vi "Real-Time Main-Final_Local_Digital.vi"() -> ()   [LabVIEW 2024]
uses:
  <vilib>/Platform/TimedLoop/XDataNode/timing_clust.ctl
  <vilib>/Platform/TimedLoop/XDataNode/nitl_modes.ctl
  <vilib>/Platform/TimedLoop/XDataNode/wakeup.ctl
  <instrlib>/niScope/Controls/niScope trigger source digital.ctl
  <instrlib>/niScope/Configure/Trigger/niScope Configure Trigger Digital.vi
  <instrlib>/niScope/Acquire/Fetch/niScope Fetch WDT.vi
  <vilib>/Waveform/WDTOps.llb/WDT Get Waveform Time Array DBL.vi
  <vilib>/platform/TimedLoop/XDataNode/XDataNode.xnode
  <vilib>/Platform/TimedLoop/XDataNode/XDNodeRunTimeDep.lvlib
panel:
  in  "channels":string="0"
  in  "FileName":string
  out "# of Chunks Fetched":i32
  out "# of Points Fetched":i32
  out "Horizontal:Actual Sample Rate":dbl
  in  "stop":bool
  in  "Fetch:Fetch Relative To":i32(ring)=482 items=["Start"=482, "Trigger"=483, "Pretrigger"=477, "Now"=481, "Read Pointer"=388]
  out "wfm":waveform(dbl)(graph)
  out "Time_shift":dbl
  in  "Resource Name":refnum<k15>="Dev1" caption="Resource Name(s)"
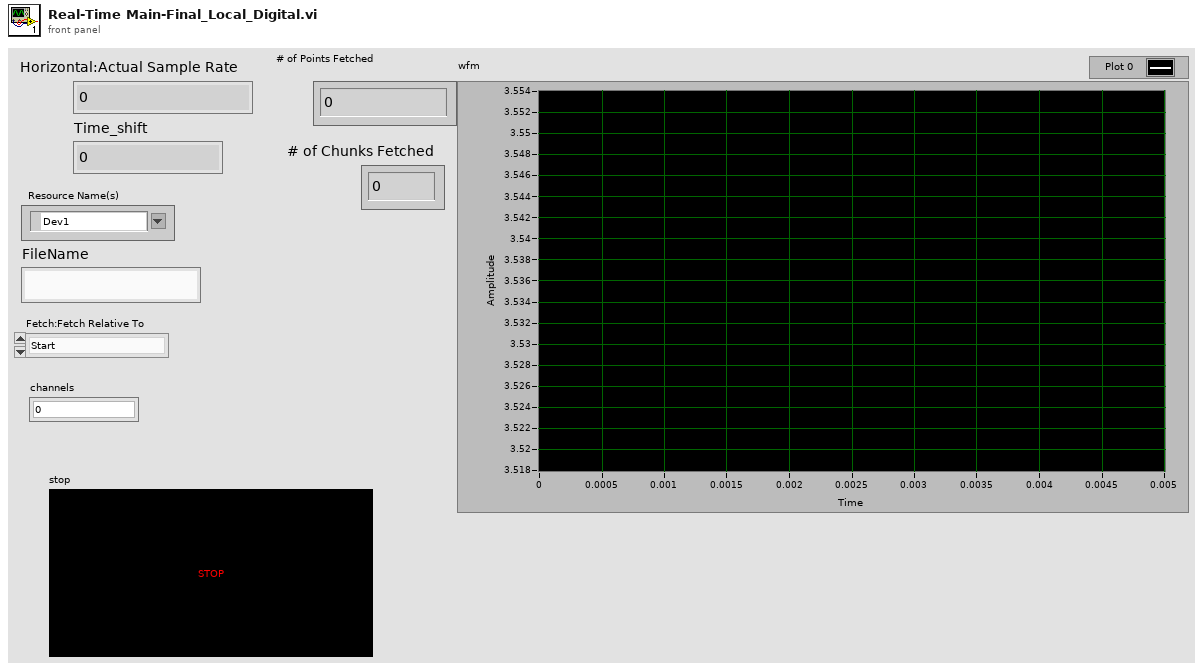
[diagram p1: front panel]
types:
  T1 = enum16{"open", "open or create", "create or replace", "create", "open (read-only)"}
  T2 = typedef "XDNodeRunTimeDep.lvlib/timing_clust.ctl" = cluster{"Expected End [f-1]":u64, "Actual End [f-1]":u64, "Finished Late? [f-1]":bool, "Expected End [i-1]":u64, "Actual End [i-1]":u64, "Finished Late? [i-1]":bool, "Expected Start [i]":u64, "Actual Start [i]":u64, "Expected Start [f]":u64, "Actual Start [f]":u64, "Source Name":string, "Structure Name":string, "Period":i64, "Deadline":i64, "Offset":i64, "Start":i64, "Priority":i32, "Timeout":i32, "Mode":T3, "Wakeup Reason":T4, "Error":errorcluster, "Source Type":string, "Secondary Source Type":string, "Global End Time":u64, "Global Start Time":u64, "Frame Duration":u64, "Iteration Duration":u64, "Assigned CPU":i32, "I/O Scan Engine Mode":u32}
  T3 = typedef "XDNodeRunTimeDep.lvlib/nitl_modes.ctl" = enum32{"No Change", "Process missed periods, maintain original phase", "Discard missed periods, maintain original phase", "Process missed periods, ignore original phase", "Discard missed periods, ignore original phase"}
  T4 = typedef "XDNodeRunTimeDep.lvlib/wakeup.ctl" = enum32{"Normal", "Aborted", "Asynchronous wakeup", "Timing source error", "Timed loop error", "Timeout"}
  T5 = typedef "niScope trigger source digital.ctl" = string
  T6 = cluster{"actualSamples":i32, "absoluteInitialX":dbl, "relativeInitialX":dbl, "xIncrement":dbl, "offset":dbl, "gain":dbl, "reserved1":dbl, "reserved2":dbl}
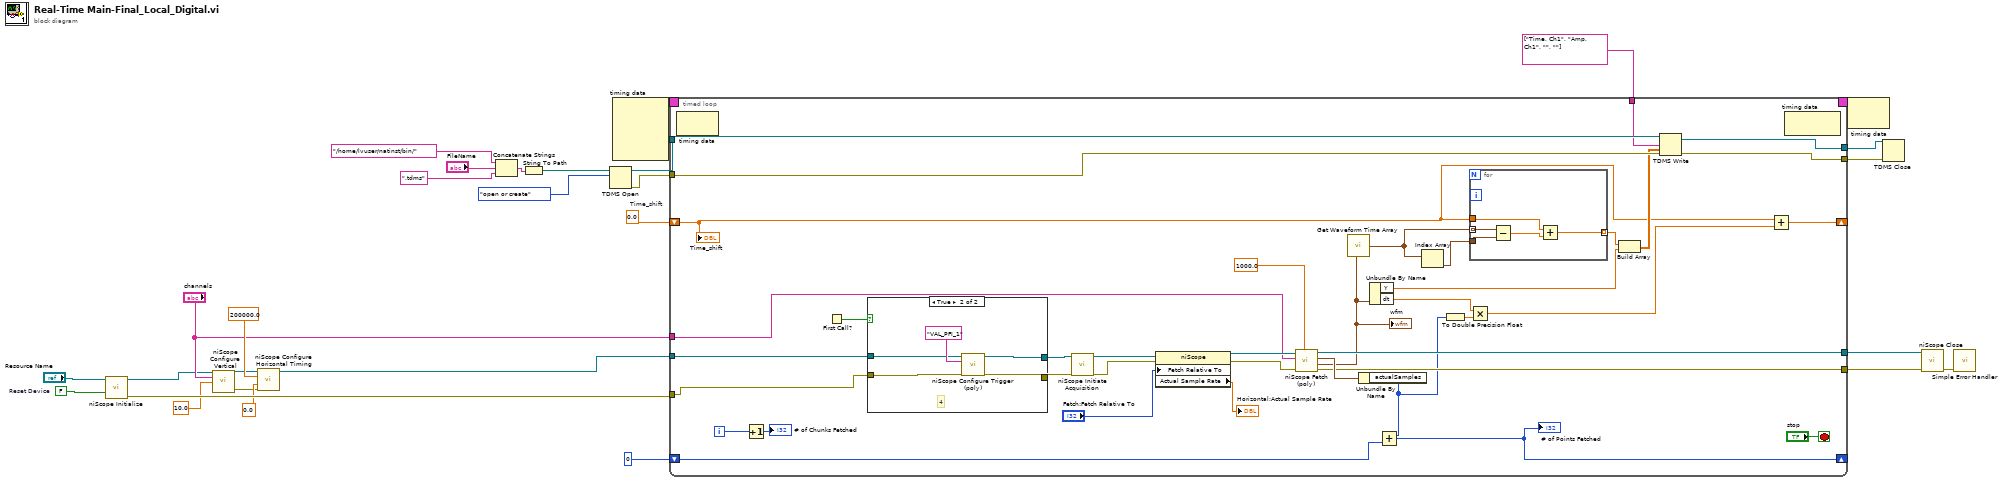
[diagram p0: block diagram]
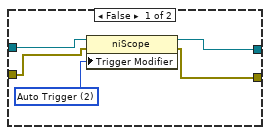
[diagram p2: hidden frame]
diagram:
  w14 = 0.0  # Time_shift
  w27 = FALSE  # Reset Device
  n1 = call <instrlib>:"niScope Initialize.vi"("resource name"="Resource Name", "reset device"=w27) -> ("instrument handle"=w2:refnum<k15>, "error out"=w21:errorcluster)  [unwired: 12 in]
  n2 = call <instrlib>:"niScope Configure Vertical.vi"("instrument handle"=w2, "channels"="channels", "vertical range"=10.0) -> ("instrument handle out"=w4:refnum<k15>, "error out"=w6:errorcluster)  [unwired: 11 in]
  n3 = call <instrlib>:"niScope Configure Horizontal Timing.vi"("instrument handle"=w4, "min sample rate"=200000.0, "reference position"=0.0, "error in"=w6) -> ("instrument handle out"=w1:refnum<k15>)  [unwired: 10 in, 1 out]
  n4 = Concatenate Strings("/home/lvuser/natinst/bin/" ("string"), "FileName", ".tdms" ("string")) -> (w13:string)
  n5 = String To Path(string=w13) -> (path=w11:path)
  n6 = TDMS Open(10:T1."open or create" ("operation (0:open)"), 11:w11) -> (0:w17:errorcluster, 3:w16:refnum<k34>)  [unwired: 5 in]
  n7 = node-c288() -> (w29:T2)  [unwired: 4 in]
  n8 = timed-loop {
    timing: w29 -> [_]
    timing-out: [_] -> w28
    tunnel: [w58] -> w25
    shift-right: [w56] -> _
    shift-left: 0 -> [w57]
    tunnel: [w46] -> w22
    tunnel: w21 -> [w33]
    tunnel: w16 -> [w51]
    tunnel: w17 -> [w50]
    tunnel: [w49] -> w19
    tunnel: [w48] -> w18
    tunnel: string[] ["Time, Ch1", "Amp, Ch1", "", ""] ("channel name(s) in (Untitled)") -> [w47]
    shift-right: [w38] -> _
    shift-left: w14 -> [w37]
    tunnel: "channels" -> [w32]
    tunnel: w1 -> [w31]
    i -> [w55]
    stop <- "stop" stop-if-true
    n9 = node-c288() -> ()  [unwired: 1 in, 1 out]
    n10 = Increment(x=w55) -> (x+1=→"# of Chunks Fetched":i32)
    n11 = First Call?() -> (First Call?: T/F=w66:bool)
    n12 = case shown="True" w66 {
      tunnel: [w76 w82] -> w67
      tunnel: [w77 w81] -> w60
      tunnel: w33 -> [w74 w80]
      tunnel: w31 -> [w73 w78]
      frame False {
        w75 = 2 items=["None"=1, "Auto Trigger"=2] ("Triggering:Trigger Modifier")
        n13 = property class="niScope"(reference=w73, error in=w74, "Trigger Modifier"=w75) -> (reference out=w77:refnum<k15>, error out=w76:errorcluster)
      }
      frame True {
        # "4"
        n14 = call-poly <instrlib>:"niScope Configure Trigger (poly).vi"("instrument handle"=w78, "trigger source"=T5 "VAL_PFI_1", "error in"=w80) -> ("instrument handle out"=w81:refnum<k15>, "error out"=w82:errorcluster)  [unwired: 11 in]
      }
    }
    n15 = call <instrlib>:"niScope Initiate Acquisition.vi"("instrument handle"=w60, "error in"=w67) -> ("instrument handle out"=w61:refnum<k15>, "error out"=w65:errorcluster)  [unwired: 12 in]
    n16 = property class="niScope"(reference=w61, error in=w65, "Fetch Relative To"="Fetch:Fetch Relative To") -> (reference out=w62:refnum<k15>, error out=w63:errorcluster, "Actual Sample Rate"=→"Horizontal:Actual Sample Rate":dbl)
    n17 = call-poly <instrlib>:"niScope Fetch (poly).vi"("timeout"=1000.0, "error in"=w63, "channels"=w32, "instrument handle"=w62) -> ("error out"=w46:errorcluster, "wfm"=w40:waveform(dbl), "wfm info"=w54:T6, "instrument handle out"=w58:refnum<k15>)  [unwired: 4 in]
    "wfm" <- w40
    n18 = call-poly <vilib>:"Get Waveform Time Array.vi"("waveform in"=w40) -> ("X array"=w41:timestamp[])  [unwired: 9 in, 1 out]
    n19 = Unbundle By Name(w54) -> ("actualSamples"=w36:i32)
    n20 = Unbundle By Name(w40) -> ("Y"=w45:dbl[], "dt"=w35:dbl)
    n21 = Add(x=w36, y=w57) -> (x+y=w56:i32)
    "# of Points Fetched" <- w56
    n22 = Index Array(array=w41) -> (element=w42:timestamp)  [unwired: 1 in]
    n23 = To Double Precision Float(number=w36) -> (double precision float=w39:dbl)
    n24 = Multiply(x=w35, y=w39) -> (x*y=w34:dbl)
    n25 = for {
      tunnel: [w70] -> w43 mode=indexing
      tunnel: w42 -> [w72]
      tunnel: w41 -> [w71] mode=indexing
      tunnel: w37 -> [w68]
      n26 = Subtract(x=w71, y=w72) -> (x-y=w69:dbl)
      n27 = Add(x=w68, y=w69) -> (x+y=w70:dbl)
    }
    n28 = Build Array(w43, w45) -> (w44:dbl[][])
    n29 = TDMS Write(0:w51, 7:w47, 9:w44, 11:w50) -> (4:w49:refnum<k34>, 15:w48:errorcluster)  [unwired: 2 in, 2 out]
    n30 = Add(x=w37, y=w34) -> (x+y=w38:dbl)
    n31 = node-c288() -> ()  [unwired: 1 in, 1 out]
    "Time_shift" <- w37
  }
  n32 = node-c288(w28) -> ()  [unwired: 1 out]
  n33 = TDMS Close(8:w18, 11:w19) -> ()  [unwired: 2 out]
  n34 = call <instrlib>:"niScope Close.vi"("instrument handle"=w25, "error in"=w22) -> ("error out"=w23:errorcluster)  [unwired: 13 in]
  n35 = call <vilib>:"Simple Error Handler.vi"("error in (no error)"=w23) -> ()  [unwired: 4 in, 5 out]
